vi "Angle_Of_Attack_in_DLR_Navigation_Reference_System (SubVI).vi"(9 "Wind Velocity":sgl[](array[numeric]), 10 "Vehicle Velocity":sgl[](array[numeric]), 11 "Quaternion":sgl[](array[numeric])) -> (2 "AoA Yaw":sgl, 3 "AoA Pitch":sgl)   [LabVIEW 2017]
uses:
  <vilib>/rvi/FXPMathLib/FxpAtan2/subVIs/nifxpmath_Atan2_SimConfig.ctl
  <vilib>/rvi/FXPMathLib/FxpAtan2/simVIs/DllFxpAtan2Temp_sub.vi
  <vilib>/rvi/FXPMathLib/FxpAtan2/XNode/nifxpmath_Atan2.xnode
panel:
  out "a 4":sgl
  out "a 3":sgl
  out "a 2":sgl
  out "a 1":sgl
  out "v":sgl[](array[numeric])
  out "r":sgl[](array[numeric])
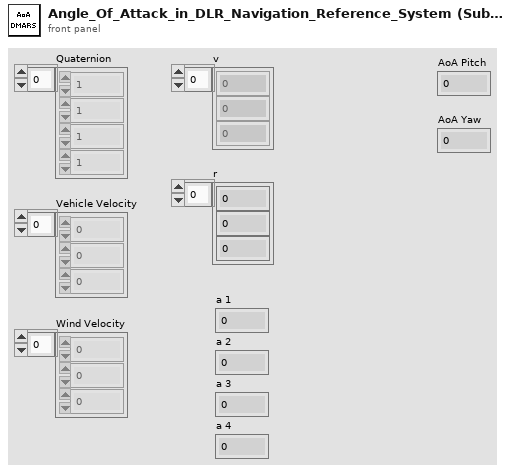
[diagram p1: front panel]
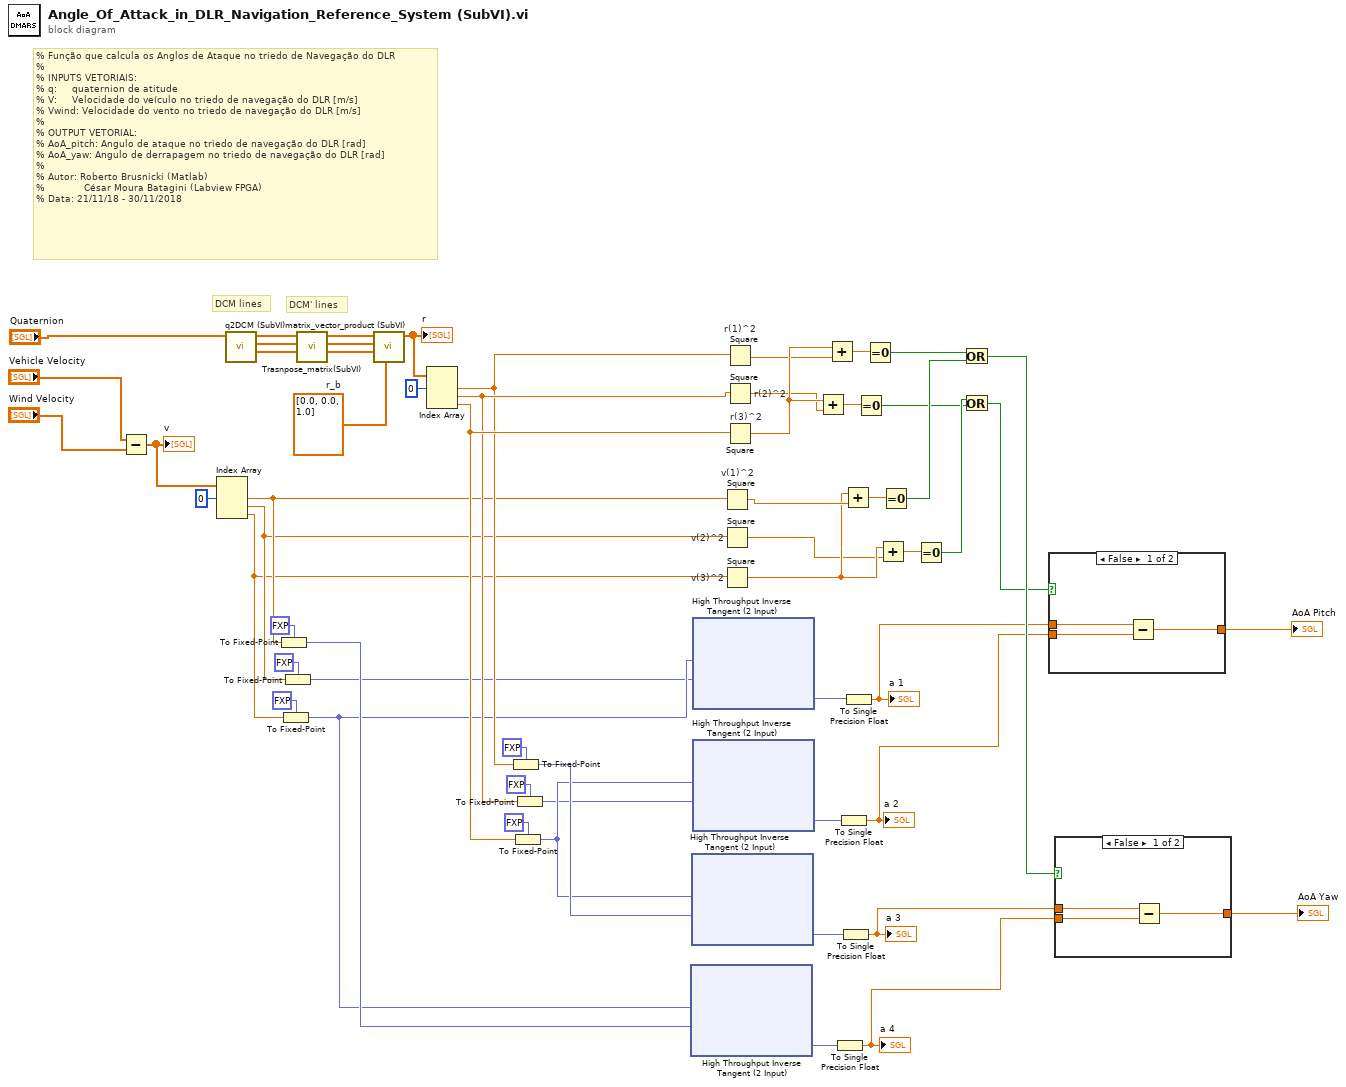
[diagram p0: block diagram]
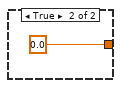
[diagram p2: hidden frame]
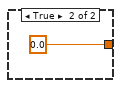
[diagram p3: hidden frame]
diagram:
  w8 = sgl[] [0.0, 0.0, 1.0]  # r_b
  # "% Função que calcula os Anglos de Ataque no triedo de Navegação do DLR \n%\n% INPUTS VETORIAIS: \n% q:     quaternion de atitude   \n% V:     Velocidade do veículo no triedo de navegação do DLR [m/s]\n% Vwind: Velocidade do vento no triedo de navegação do DLR [m/s]\n%\n% OUTPUT VETORIAL:\n% AoA_pitch: Angulo de ataque no triedo de navegação do DLR [rad]\n% AoA_yaw: Angulo de derrapagem no triedo de navegação do DLR [rad]\n%\n% Autor: Roberto Brusnicki (Matlab)\n%             César Moura Batagini (Labview FPGA)\n% Data: 21/11/18 - 30/11/2018"
  # "DCM' lines"
  # "DCM lines"
  n1 = Subtract(x="Vehicle Velocity", y="Wind Velocity") -> (x-y=w12:sgl[])
  "v" <- w12
  n2 = Index Array(array=w12, index #1=0 ("index")) -> (element #1=w33:sgl, element #2=w32:sgl, element #3=w31:sgl)  [unwired: 2 in]
  n3 = call "q2DCM (SubVI).vi"("Quaternion"="Quaternion") -> ("DCM line 3"=w4:sgl[], "DCM line 2"=w3:sgl[], "DCM line 1"=w2:sgl[])  [unwired: 8 in]
  n4 = To Fixed-Point(fixed-point type=fxp<+/-,16,1> 0.0 ("y"), number=w33) -> (fixed-point=w30:fxp<+/-,16,1>)
  n5 = To Fixed-Point(fixed-point type=fxp<+/-,16,1> 0.0 ("y"), number=w31) -> (fixed-point=w29:fxp<+/-,16,1>)
  n6 = To Fixed-Point(fixed-point type=fxp<+/-,16,1> 0.0 ("y"), number=w32) -> (fixed-point=w21:fxp<+/-,16,1>)
  n7 = call "Trasnpose_matrix(SubVI).vi"("Line 3"=w4, "Line 2"=w3, "Line 1"=w2) -> ("Line 3 transpose"=w7:sgl[], "Line 2 transpose"=w6:sgl[], "Line 1 transpose"=w5:sgl[])  [unwired: 6 in]
  n8 = call "matrix_vector_product (SubVI).vi"("Input vector"=w8, "Line 3"=w7, "Line 2"=w6, "Line 1"=w5) -> ("Output vector"=w20:sgl[])  [unwired: 7 in]
  "r" <- w20
  n9 = Index Array(array=w20, index #1=0 ("index")) -> (element #1=w34:sgl, element #2=w35:sgl, element #3=w36:sgl)  [unwired: 2 in]
  n10 = To Fixed-Point(fixed-point type=fxp<+/-,16,1> 0.0 ("y"), number=w34) -> (fixed-point=w28:fxp<+/-,16,1>)
  n11 = To Fixed-Point(fixed-point type=fxp<+/-,16,1> 0.0 ("y"), number=w36) -> (fixed-point=w27:fxp<+/-,16,1>)
  n12 = To Fixed-Point(fixed-point type=fxp<+/-,16,1> 0.0 ("y"), number=w35) -> (fixed-point=w26:fxp<+/-,16,1>)
  n13 = xnode "High Throughput Inverse Tangent (2 Input)"("y"=w29, "x"=w30) -> ("atan2(y,x) (pi)"=w25:fxp<+/-,16,2>)
  n14 = xnode "High Throughput Inverse Tangent (2 Input)"("y"=w27, "x"=w28) -> ("atan2(y,x) (pi)"=w24:fxp<+/-,16,2>)
  n15 = xnode "High Throughput Inverse Tangent (2 Input)"("y"=w29, "x"=w21) -> ("atan2(y,x) (pi)"=w22:fxp<+/-,16,2>)
  n16 = xnode "High Throughput Inverse Tangent (2 Input)"("y"=w27, "x"=w26) -> ("atan2(y,x) (pi)"=w23:fxp<+/-,16,2>)
  n17 = Square "v(1)^2"(x=w33) -> (x^2=w53:sgl)
  n18 = Square "v(2)^2"(x=w32) -> (x^2=w37:sgl)
  n19 = Square "v(3)^2"(x=w31) -> (x^2=w52:sgl)
  n20 = Square "r(1)^2"(x=w34) -> (x^2=w49:sgl)
  n21 = Square "r(2)^2"(x=w35) -> (x^2=w40:sgl)
  n22 = Square "r(3)^2"(x=w36) -> (x^2=w50:sgl)
  n23 = Add(x=w50, y=w40) -> (x+y=w39:sgl)
  n24 = Add(x=w50, y=w49) -> (x+y=w47:sgl)
  n25 = To Single Precision Float(number=w25) -> (single precision float=w58:sgl)
  "a 4" <- w58
  n26 = To Single Precision Float(number=w23) -> (single precision float=w46:sgl)
  "a 2" <- w46
  n27 = To Single Precision Float(number=w24) -> (single precision float=w57:sgl)
  "a 3" <- w57
  n28 = Add(x=w52, y=w53) -> (x+y=w48:sgl)
  n29 = To Single Precision Float(number=w22) -> (single precision float=w45:sgl)
  "a 1" <- w45
  n30 = Equal To 0?(x=w39) -> (x = 0?=w41:bool)
  n31 = Equal To 0?(x=w47) -> (x = 0?=w51:bool)
  n32 = Add(x=w52, y=w37) -> (x+y=w38:sgl)
  n33 = Equal To 0?(x=w48) -> (x = 0?=w54:bool)
  n34 = Equal To 0?(x=w38) -> (x = 0?=w42:bool)
  n35 = Or(x=w51, y=w54) -> (x .or. y?=w56:bool)
  n36 = Or(x=w42, y=w41) -> (x .or. y?=w43:bool)
  n37 = case shown="False" w43 {
    tunnel: [w59 sgl 0.0] -> w44
    tunnel: w45 -> [w61 _]
    tunnel: w46 -> [w60 _]
    frame False {
      n38 = Subtract(x=w61, y=w60) -> (x-y=w59:sgl)
    }
    frame True {
    }
  }
  "AoA Pitch" <- w44
  n39 = case shown="False" w56 {
    tunnel: [w63 sgl 0.0] -> w55
    tunnel: w57 -> [w65 _]
    tunnel: w58 -> [w64 _]
    frame False {
      n40 = Subtract(x=w65, y=w64) -> (x-y=w63:sgl)
    }
    frame True {
    }
  }
  "AoA Yaw" <- w55
